vi "LabVIEW_Basic_Serial_Arduino.vi"() -> ()   [LabVIEW 2020]
uses:
  <vilib>/Instr/_visa.llb/Select Event Type.ctl
  <vilib>/Instr/_visa.llb/VISA Configure Serial Port (Instr).vi
panel:
  in  "Stop":bool
  in  "Tab Control":T1(tab)
  out "Serial Read Buffer":string
  in  "VISA resource name":refnum<visa-resource-name>="COM17"
  in  "baud rate (9600)":u32=9600
  in  "Time Target (s)":dbl=1.0
  out "Elapsed Time (s)":dbl
  # "Basic Serial Communication Between LabVIEW and Arduino"
  # "Auther: Suparat Yeamkuan\nOverview: Demonstrates the use of serial communication between LabVIEW and Arduino.\nRequirements: Arduino UNO and  NI-VISA Driver."
  # "Instructions:\n1. Connect USB cable from Arduino board to computer.\n2. Use Arduino IDE to upload the code to Arduino board."
  # "Instructions:\n1. Select the VISA resource name as a COM port that Arduino connect to computer, this can show the COM port device manager.\n2. Run the VI.\n3. If your Arduino is send message back, it will display in \"Serial Read Buffer\"."
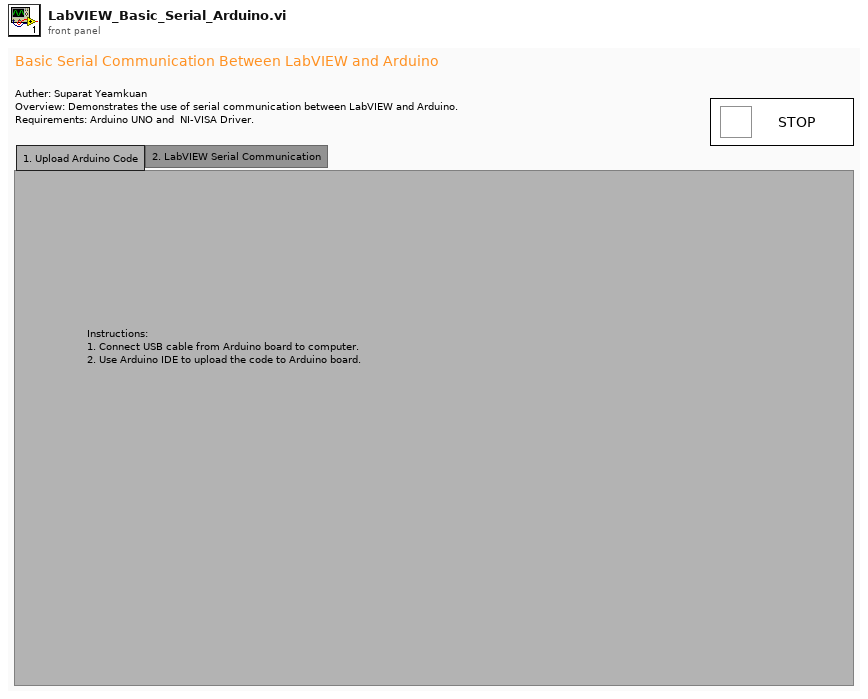
[diagram p1: front panel]
types:
  T1 = enum32{"1. Upload Arduino Code", "2. LabVIEW Serial Communication"}
  T2 = typedef "Select Event Type.ctl" = u32
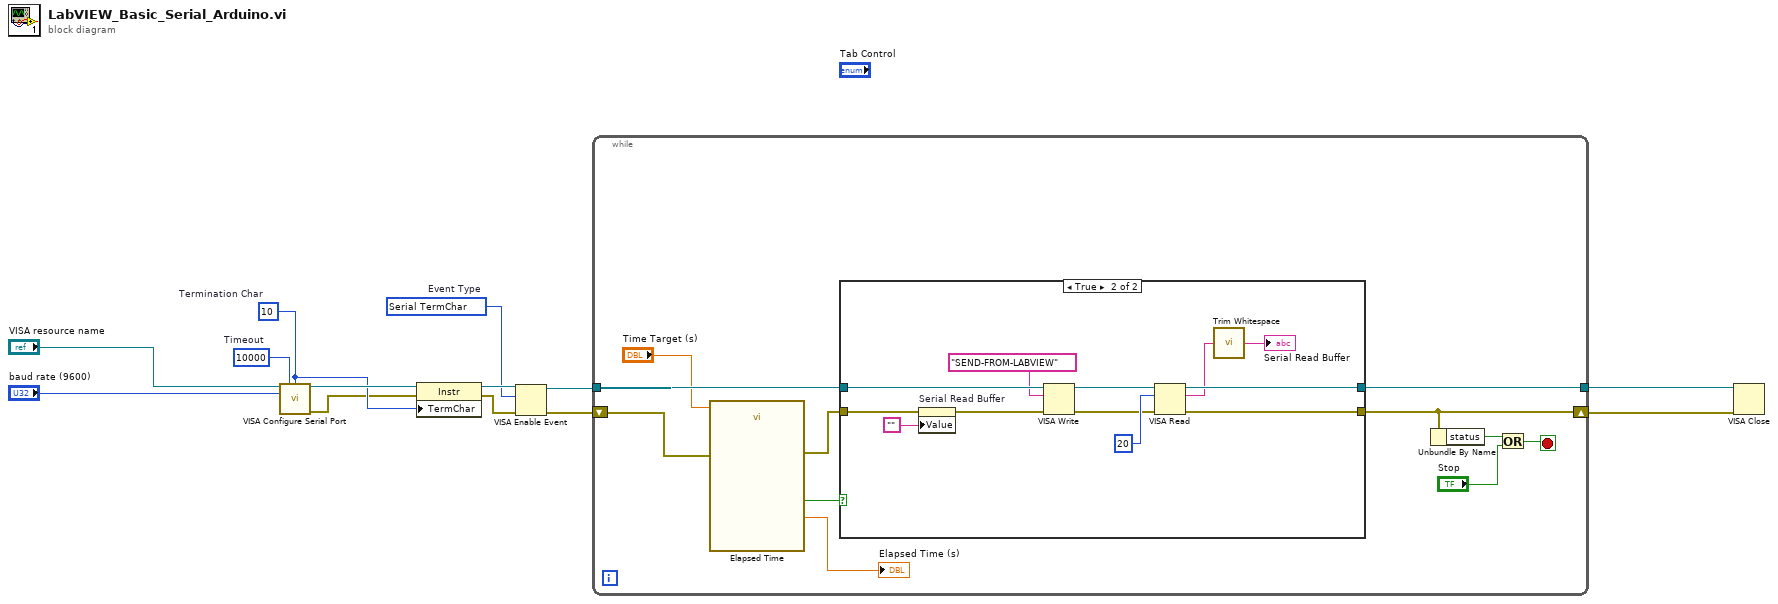
[diagram p0: block diagram]
diagram:
  w5 = T2 1073684516 items=["Service Request"=1073684491, "Trigger"=3221168138, "Clear"=1073684493, "VXI Signal"=1073684512, "VXI/VME Interrupt"=3221168161, "VXI/VME Sysfail"=1073684509, "VXI/VME Sysreset"=1073684510, "GPIB CIC"=1073684498, "GPIB Talk"=1073684499, "GPIB Listen"=1073684500, "PXI Interrupt"=1073684514, "Serial Break"=1073684515, "Serial TermChar"=1073684516, "Serial CTS"=1073684521, "Serial DSR"=1073684522, "Serial DCD"=1073684524, "Serial RI"=1073684526, "Serial Character"=1073684533, "USB Interrupt"=1073684535, "All Enabled"=1073709055]  # Event Type
  w9 = u8 10  # Termination Char
  w11 = u32 10000  # Timeout
  n1 = call-poly "VISA Configure Serial Port"("VISA resource name"="VISA resource name", "timeout (10sec)"=w11, "termination char\n(0xA = '\\n' = LF)"=w9, "baud rate (9600)"="baud rate (9600)") -> ("VISA resource name out"=w10:refnum<visa-resource-name>, "error out"=w8:errorcluster)  [unwired: 10 in]
  n2 = property class="Instr"(reference=w10, error in=w8, "TermChar"=w9) -> (reference out=w7:refnum<visa-resource-name>, error out=w6:errorcluster)
  n3 = VISA Enable Event(8:w6, 10:w5, 11:w7) -> (0:w4:errorcluster, 3:w3:refnum<visa-resource-name>)  [unwired: 1 in]
  n4 = while {
    shift-right: [w23] -> w12
    shift-left: w4 -> [w17]
    tunnel: [w24] -> w13
    tunnel: w3 -> [w19]
    stop <- w21 stop-if-true
    n5 = call "Elapsed Time"("Time Target (s)"="Time Target (s)", "error in (no error)"=w17) -> ("Elapsed Time (s)"=→"Elapsed Time (s)":dbl, "Time has Elapsed"=w18:bool, "error out"=w16:errorcluster)  [unwired: 10 in, 5 out]
    n6 = case shown="True" w18 {
      tunnel: [w26 w38] -> w24
      tunnel: [w25 w37] -> w23
      tunnel: w19 -> [w26 w33]
      tunnel: w16 -> [w25 w29]
      frame False {
      }
      frame True {
        n7 = property on="Serial Read Buffer" class="Str"(error in=w29, "Value"="") -> (error out=w28:errorcluster)  [unwired: 1 in, 1 out]
        n8 = VISA Write(VISA resource name=w33, write buffer="SEND-FROM-LABVIEW", error in (no error)=w28) -> (VISA resource name out=w32:refnum<visa-resource-name>, error out=w31:errorcluster)  [unwired: 1 out]
        n9 = VISA Read(VISA resource name=w32, byte count=u32 20, error in (no error)=w31) -> (VISA resource name out=w38:refnum<visa-resource-name>, read buffer=w35:string, error out=w37:errorcluster)  [unwired: 1 out]
        n10 = call <vilib>:"Trim Whitespace.vi"("string"=w35) -> ("trimmed string"=→"Serial Read Buffer":string)  [unwired: 1 in]
      }
    }
    n11 = Unbundle By Name(w23) -> ("status"=w22:bool)
    n12 = Or(x=w22, y="Stop") -> (x .or. y?=w21:bool)
  }
  n13 = VISA Close(VISA resource name=w13, error in (no error)=w12) -> ()  [unwired: 1 out]
